vi "Calc Inputs.vi"(8 "error in (no error)":errorcluster, 11 "Div Calc in":refnum<class "Div Calc.lvclass">) -> (0 "error out":errorcluster, 2 "Inputs":string[](array[string]))   [LabVIEW 2020, in "VolatusCalcs.lvlib" / "Div Calc.lvclass"]
uses:
  Div Calc.lvclass
  Div Calc.lvclass/Div Calc.ctl
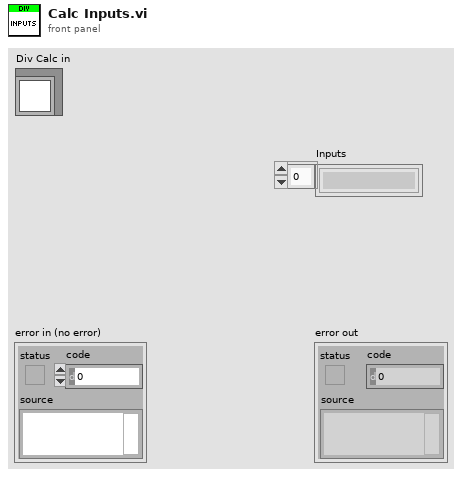
[diagram p1: front panel]
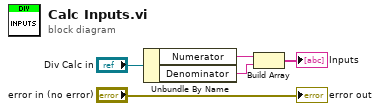
[diagram p0: block diagram]
diagram:
  n1 = Unbundle By Name("Div Calc in") -> ("Numerator"=w3:string, "Denominator"=w2:string)
  n2 = Build Array(w3, w2) -> (→"Inputs":string[])
  "error out" <- "error in (no error)"
